vi "NameFileFromTimestamp.vi"(11 "TimeStampData":cluster{"time":string}) -> (3 "String":string)   [LabVIEW 2019]
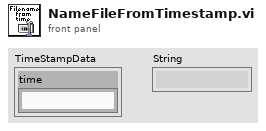
[diagram p1: front panel]
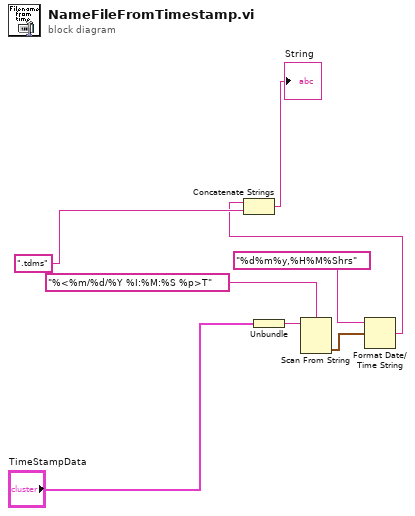
[diagram p0: block diagram]
diagram:
  n1 = Unbundle("TimeStampData") -> ("time"=w3:string)
  n2 = Scan From String(format string="%<%m/%d/%Y %I:%M:%S %p>T", input string=w3) -> (output 1=w5:timestamp)  [unwired: 3 in, 3 out]
  n3 = Format Date/Time String(time format string (%c)="%d%m%y,%H%M%Shrs", seconds (now)=w5) -> (date/time string=w7:string)  [unwired: 1 in]
  n4 = Concatenate Strings(w7, ".tdms") -> (→"String":string)
